vi "Actor Core.vi"(8 "error in":errorcluster, 11 "Nested in":refnum<class "Generador funciones ACQ.lvclass">) -> (0 "error out":errorcluster, 3 "Actor out":refnum<class "Actor.lvclass">)   [LabVIEW 2019, in "Generador funciones ACQ.lvlib" / "Generador funciones ACQ.lvclass"]
doc: "(<B>Filename</B>: Actor Framework.lvlib:Actor.lvclass:Actor Core.vi)\n\nReceives messages to the actor, reacts to them, and initiates any error handling that may shut the actor down.\n\nDescendant classes may override this VI to append parallel tasks for the actor to complete while it handles messages. Overrides use the Call Parent Method node."
uses:
  Generador funciones ACQ.lvclass
  C:/Program Files/National Instruments/LabVIEW 2019/vi.lib/ActorFramework/Actor/Actor.lvclass
  <vilib>/ActorFramework/Actor/Actor.lvclass
  <vilib>/ActorFramework/Actor/Actor.lvclass/Actor.ctl
  Generador funciones ACQ.lvclass/Generador funciones ACQ.ctl
  Generador funciones Messages/Graph Data Msg/Graph Data Msg.lvclass/Graph Data Msg.ctl
  <vilib>/ActorFramework/Message Enqueuer/Message Enqueuer.lvclass/Message Enqueuer.ctl
  Generador funciones Messages/Datos grafica Msg/Datos grafica Msg.lvclass/Datos grafica Msg.ctl
  <vilib>/ActorFramework/Message Enqueuer/Enqueue.vi
  <vilib>/Utility/error.llb/Clear Errors.vi
  Generador funciones Messages/Datos grafica Msg/Datos grafica Msg.lvclass
  C:/Program Files/National Instruments/LabVIEW 2019/vi.lib/ActorFramework/Message/Message.lvclass
  Generador funciones Messages/Graph Data Msg/Graph Data Msg.lvclass
  <vilib>/ActorFramework/Stop Msg/Stop Msg.lvclass
  <vilib>/ActorFramework/Message Priority Queue/Priority Enqueue.vi
  <vilib>/measure/NI_MABase.lvlib
  <vilib>/Analysis/NI_AALBase.lvlib
panel:
  out "Numeric Control":dbl
  out "Waveform Chart":waveform(dbl)(graph)
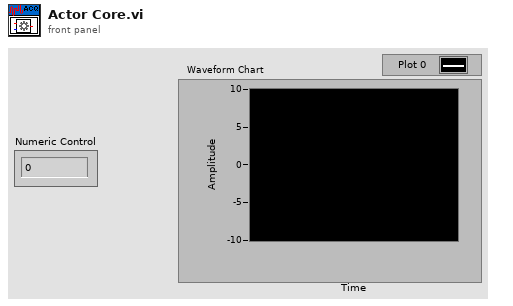
[diagram p1: front panel]
types:
  T1 = cluster{"Stop":refnum<user-event>, "Frecuencia":refnum<user-event>, "Amplitud":refnum<user-event>, "Start/Stop":refnum<user-event>, "Tipo de señal":refnum<user-event>}
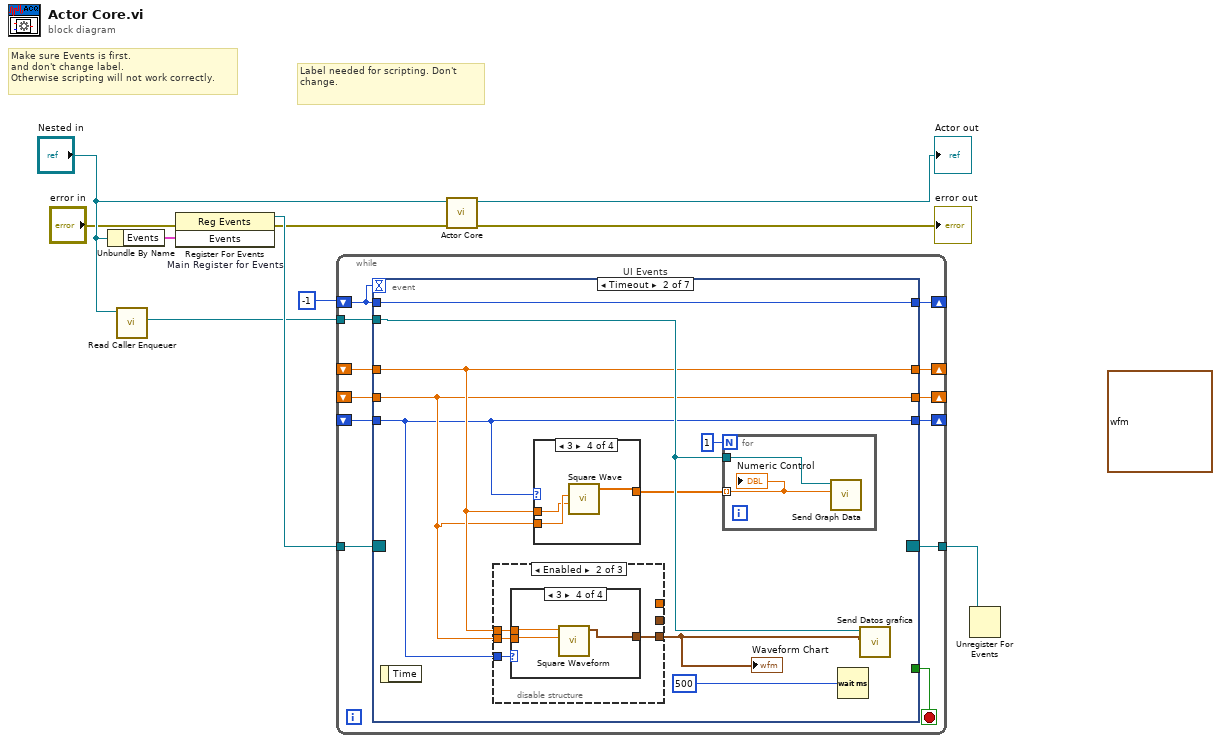
[diagram p0: block diagram]
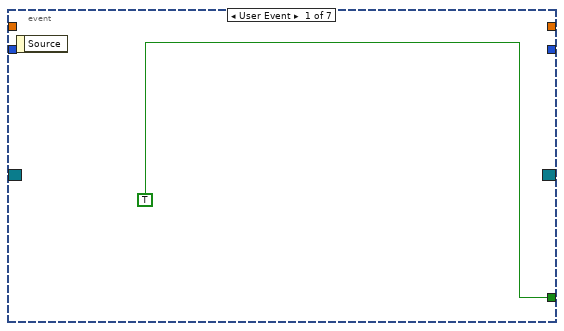
[diagram p2: hidden frame]
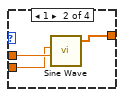
[diagram p4: hidden frame]
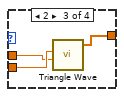
[diagram p5: hidden frame]
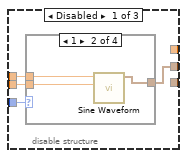
[diagram p6: hidden frame]
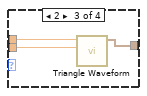
[diagram p8: hidden frame]
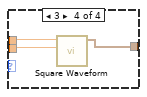
[diagram p9: hidden frame]
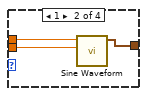
[diagram p11: hidden frame]
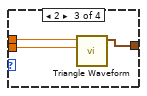
[diagram p12: hidden frame]
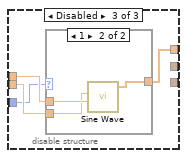
[diagram p13: hidden frame]
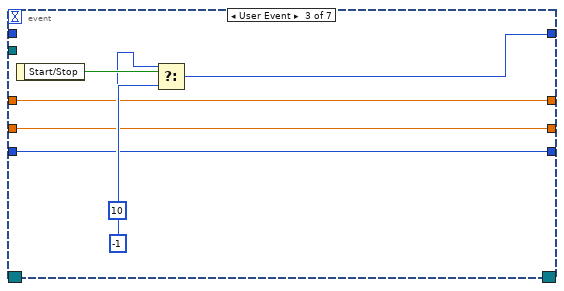
[diagram p15: hidden frame]
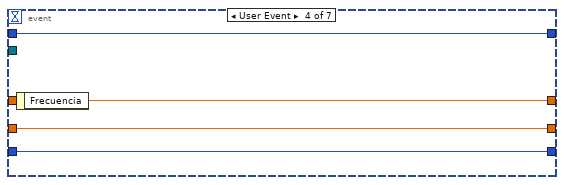
[diagram p16: hidden frame]
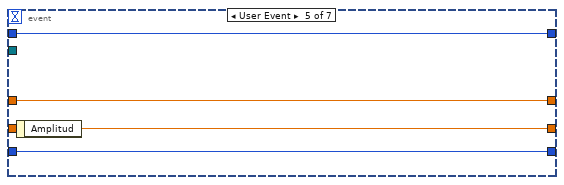
[diagram p17: hidden frame]
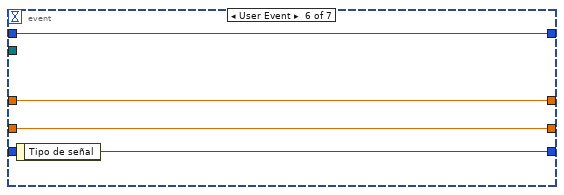
[diagram p18: hidden frame]
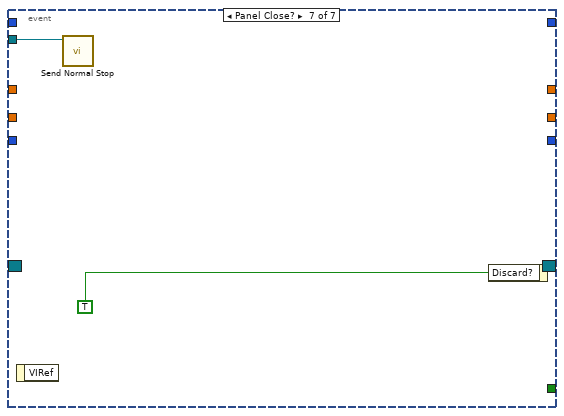
[diagram p19: hidden frame]
diagram:
  (unwired) waveform(dbl) {"t0"=timestamp(0 s since 1904-01-01), "dt"=1.0, "Y"=[]} ("Waveform")
  # "Label needed for scripting. Don't change."
  # "Make sure Events is first.\nand don't change label.\nOtherwise scripting will not work correctly."
  n1 = Unbundle By Name("Nested in") -> ("Events"=w7:T1)
  n2 = call <vilib>:"Read Caller Enqueuer.vi"("Actor"="Nested in") -> ("Caller Enqueuer"=w4:refnum<class "Message Enqueuer.lvclass">)  [unwired: 10 in]
  n3 = register-events "Main Register for Events"(error in="error in", w7) -> (reference out=w8:refnum<event-registration>, error out=w2:errorcluster)  [unwired: 1 in]
  n4 = while {
    tunnel: w8 -> [w22]
    tunnel: [w20] -> w6
    tunnel: w4 -> [w19]
    shift-right: [w18] -> _
    shift-left: -1 -> [w17]
    shift-right: [w16] -> _
    shift-left: _ -> [w15]
    shift-right: [w14] -> _
    shift-left: _ -> [w13]
    shift-right: [w12] -> _
    shift-left: _ -> [w11]
    stop <- w21 stop-if-true
    n5 = event "UI Events" shown="[1] Timeout" {
      selector: w22 -> [_ _ _ _ _ _ _]
      dyn-events: [_ _ _ _ _ _ _] -> w20
      timeout: w17 -> [_ _ _ _ _ _ _]
      tunnel: [TRUE _ _ _ _ _ _] -> w21
      tunnel: w19 -> [_ w29 _ _ _ _ w96]
      tunnel: [_ w32 w82 w87 w91 w95 _] -> w18
      tunnel: w17 -> [_ w32 _ w87 w91 w95 _]
      tunnel: [_ w27 w79 w86 w90 w94 _] -> w16
      tunnel: w15 -> [_ w27 w79 _ w90 w94 _]
      tunnel: [_ w26 w78 w84 w89 w93 _] -> w14
      tunnel: w13 -> [_ w26 w78 w84 _ w93 _]
      tunnel: [_ w25 w77 w85 w88 w92 _] -> w12
      tunnel: w11 -> [_ w25 w77 w85 w88 _ _]
      event User Event {
        n6 = event-data() -> ()  [unwired: 1 in, 1 out]
      }
      event Timeout {
        n7 = event-data() -> ()  [unwired: 1 in, 1 out]
        n8 = disable-structure shown="Enabled" {
          disable-tunnel: w25 -> [w47 w60 w71]
          disable-tunnel: w27 -> [w46 w59 w73]
          disable-tunnel: w26 -> [w45 w58 w72]
          disable-tunnel: [_ w57 _] -> w31
          disable-tunnel: [_ _ w70] -> _
          disable-tunnel: [w44 _ _] -> _
          frame Disabled {
            n9 = case shown="1" w47 {
              tunnel: w46 -> [_ w50 w53 w56]
              tunnel: w45 -> [_ w49 w52 w55]
              tunnel: [_ w48 w51 w54] -> w44
              frame 0, Default {
              }
              frame 1 {
                n10 = call <vilib>:"Sine Waveform.vi"("amplitude"=w49, "frequency"=w50) -> ("signal out"=w48:waveform(dbl))  [unwired: 8 in, 1 out]
              }
              frame 2 {
                n11 = call <vilib>:"Triangle Waveform.vi"("amplitude"=w52, "frequency"=w53) -> ("signal out"=w51:waveform(dbl))  [unwired: 8 in, 1 out]
              }
              frame 3 {
                n12 = call <vilib>:"Square Waveform.vi"("amplitude"=w55, "frequency"=w56) -> ("signal out"=w54:waveform(dbl))  [unwired: 8 in, 1 out]
              }
            }
          }
          frame Enabled {
            n13 = case shown="3" w60 {
              tunnel: w59 -> [_ w63 w66 w69]
              tunnel: w58 -> [_ w62 w65 w68]
              tunnel: [_ w61 w64 w67] -> w57
              frame 0, Default {
              }
              frame 1 {
                n14 = call <vilib>:"Sine Waveform.vi"("amplitude"=w62, "frequency"=w63) -> ("signal out"=w61:waveform(dbl))  [unwired: 8 in, 1 out]
              }
              frame 2 {
                n15 = call <vilib>:"Triangle Waveform.vi"("amplitude"=w65, "frequency"=w66) -> ("signal out"=w64:waveform(dbl))  [unwired: 8 in, 1 out]
              }
              frame 3 {
                n16 = call <vilib>:"Square Waveform.vi"("amplitude"=w68, "frequency"=w69) -> ("signal out"=w67:waveform(dbl))  [unwired: 8 in, 1 out]
              }
            }
          }
          frame Disabled {
            n17 = case shown="1" w71 {
              tunnel: w73 -> [_ w76]
              tunnel: w72 -> [_ w75]
              tunnel: [_ w74] -> w70
              frame 0, Default {
              }
              frame 1 {
                n18 = call <vilib>:"Sine Wave.vi"("amplitude"=w75, "frequency"=w76) -> ("sine wave"=w74:dbl[])  [unwired: 3 in, 2 out]
              }
            }
          }
        }
        "Waveform Chart" <- w31
        n19 = case shown="3" w25 {
          tunnel: w27 -> [_ w35 w37 w40]
          tunnel: w26 -> [_ w34 w38 w41]
          tunnel: [_ w33 w36 w39] -> w24
          frame 0, Default {
          }
          frame 1 {
            n20 = call <vilib>:"Sine Wave.vi"("amplitude"=w34, "frequency"=w35) -> ("sine wave"=w33:dbl[])  [unwired: 3 in, 2 out]
          }
          frame 2 {
            n21 = call <vilib>:"Triangle Wave.vi"("amplitude"=w38, "frequency"=w37) -> ("triangle wave"=w36:dbl[])  [unwired: 3 in, 2 out]
          }
          frame 3 {
            n22 = call <vilib>:"Square Wave.vi"("amplitude"=w41, "frequency"=w40) -> ("square wave"=w39:dbl[])  [unwired: 4 in, 2 out]
          }
        }
        n23 = for {
          N: 1 -> [_]
          tunnel: w29 -> [w43]
          tunnel: w24 -> [w42] mode=indexing
          n24 = call "Send Graph Data.vi"("Graph data"=w42, "Message Enqueuer"=w43) -> ()  [unwired: 8 in, 2 out]
          "Numeric Control" <- w42
        }
        n25 = Wait (ms)(milliseconds to wait=u32 500) -> ()  [unwired: 1 out]
        n26 = call "Send Datos grafica.vi"("Waveform"=w31, "Message Enqueuer"=w29) -> ()  [unwired: 8 in, 2 out]
      }
      event User Event {
        n27 = event-data() -> ("Start/Stop"=w83:bool)  [unwired: 1 in]
        n28 = Select(t=10, s=w83, f=-1) -> (s? t:f=w82:i32)
      }
      event User Event {
        n29 = event-data() -> ("Frecuencia"=w86:dbl)  [unwired: 1 in]
      }
      event User Event {
        n30 = event-data() -> ("Amplitud"=w89:dbl)  [unwired: 1 in]
      }
      event User Event {
        n31 = event-data() -> ("Tipo de señal"=w92:u16)  [unwired: 1 in]
      }
      event Panel Close? {
        n32 = event-data() -> ()  [unwired: 1 in, 1 out]
        n33 = call <vilib>:"Send Normal Stop.vi"("Message Enqueuer"=w96) -> ()  [unwired: 10 in, 1 out]
        n34 = event-data("Discard?"=TRUE) -> ()  [unwired: 1 in, 1 out]
      }
    }
  }
  n35 = call-parent "Actor Core.vi"("error in"=w2, "Actor in"="Nested in") -> ("error out"=→"error out":errorcluster, "Actor out"=→"Actor out":refnum<class "Actor.lvclass">)  [unwired: 8 in]
  n36 = Unregister For Events(event registration refnum=w6) -> ()  [unwired: 1 in, 1 out]
